vi "writeToXML.vi"(8 "error in (no error)":errorcluster, 10 "ClassLabel":string, 11 "TCSMCCCommand in":refnum<class "TCSMCCCommand.lvclass">) -> (0 "error out":errorcluster, 2 "XMLout":string, 3 "TCSMCCCommand out":refnum<class "TCSMCCCommand.lvclass">)   [LabVIEW 2014, in "TCSDataDefinitions.lvlib" / "TCSMountControlCommand.lvlib" / "TCSMCCCommand.lvclass"]
uses:
  TCSMCCCommand.lvclass
  TCSCommand/TCSCommand/TCSCommand.lvclass
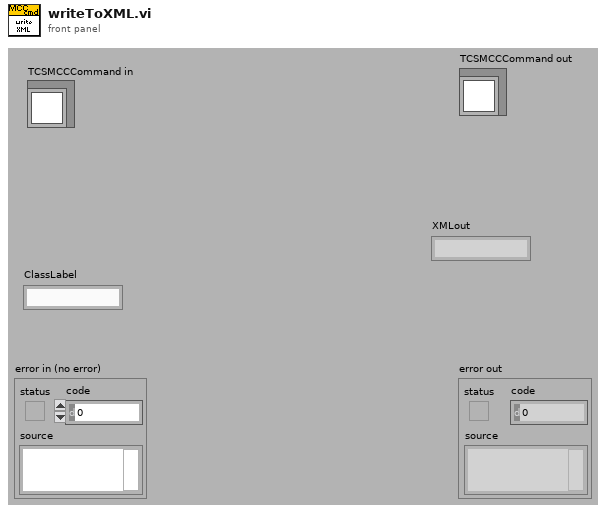
[diagram p1: front panel]
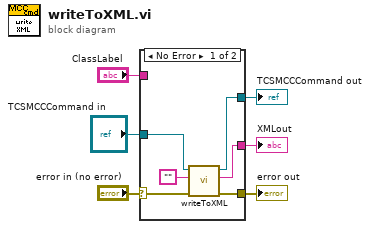
[diagram p0: block diagram]
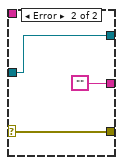
[diagram p2: hidden frame]
diagram:
  n1 = case shown="No Error" "error in (no error)" {
    selector: "error in (no error)" -> [w8 w15]
    tunnel: [w7 w15] -> w5
    tunnel: [w9 w14] -> w4
    tunnel: "TCSMCCCommand in" -> [w10 w14]
    tunnel: [w12 ""] -> w3
    tunnel: "ClassLabel" -> [_ _]
    frame No Error {
      n2 = call-parent "writeToXML.vi"("error in (no error)"=w8, "Class Label"="", "TCSCommand in"=w10) -> ("error out"=w7:errorcluster, "XML out"=w12:string, "TCSCommand out"=w9:refnum<class "TCSMCCCommand.lvclass">)  [unwired: 6 in]
    }
    frame Error {
    }
  }
  "error out" <- w5
  "TCSMCCCommand out" <- w4
  "XMLout" <- w3
